vi "Clear_Info.vi"(8 "error in (no error)":errorcluster, 11 "Class in":refnum<class "IB_MSI.lvclass">) -> (0 "error out":errorcluster, 3 "Class out":refnum<class "IB_MSI.lvclass">)   [LabVIEW 2020, in "IB_MSI.lvclass"]
uses:
  <vilib>/AppBuilder/IB_Classes/MSI/IB_MSI.lvclass
  <vilib>/AppBuilder/IB_Classes/MSI/IB_MSI.lvclass/IB_MSI.ctl
  <vilib>/AppBuilder/IB_RW_Project/IB_RW_Project_PropBag_Action.ctl
  <vilib>/AppBuilder/IB_Classes/Installer/Installer.lvclass
  e:/builds/penguin/labview/branches/2020/dev/dist/vi.lib/AppBuilder/IB_Classes/Installer/Installer.lvclass
  e:/builds/penguin/labview/branches/2020/dev/dist/vi.lib/AppBuilder/IB_Classes/MSI/IB_MSI.lvclass
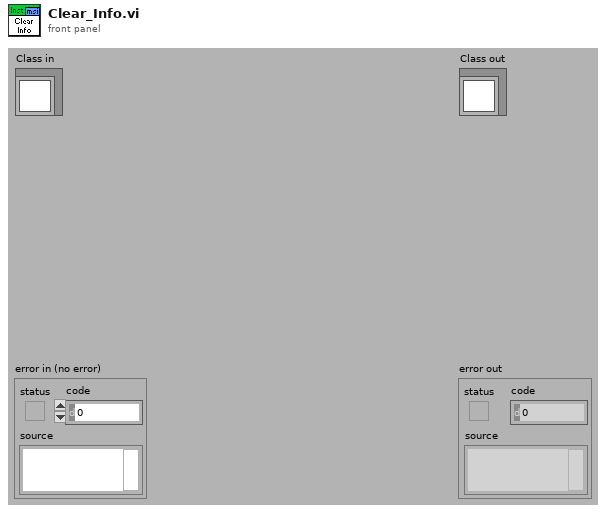
[diagram p1: front panel]
types:
  T1 = typedef "IB_RW_Project_PropBag_Action.ctl" = enum16{"read", "write", "clear", "readPrevious", "writePrevious", "clearPrevious"}
  T2 = typedef "IB_Installer.ctl" = cluster{"Destination":refnum<class "IB_Destination.lvclass">[], "Source":refnum<class "IB_Source.lvclass">[], "buildObject":T3, "defaultDir":string, "platform":string, "author":string, "productName":string, "buildSpecName":string, "hide":bool, "requireLVDevSys":bool, "autoIncrement":bool, "includeError":bool, "readmeID":string, "buildLocation":path, "readmePath":path, "mediaSize":u16, "language":T4, "productVersion":T5, "preview":bool, "programmatic":bool, "progressBarEvents":T6, "userLog_Path":path, "shortcutAddresses":T8[], "EXE_Install Address":string, "EXE_Uninstall Address":string, "additional NIPaths":refnum<class "Dest_NI_NIPath.lvclass">[], "web service itemIDs":string[], "installerName":string}
  T3 = typedef "ItemRef.ctl" = u64
  T4 = typedef "CDK_sTypeDef_Languages.ctl" = u16
  T5 = typedef "CDK_sTypeDef_ProductVersion.ctl" = cluster{"Major":u8, "Minor":u8, "Update":u16}
  T6 = typedef "provcom_ProgressBar_Events.ctl" = cluster{"newJob":refnum<user-event>, "newItem":refnum<user-event>, "errorMsg":T7, "cancel":refnum<user-event>}
  T7 = typedef "mxLvBuildError.ctl" = refnum<user-event>
  T8 = typedef "CDK_sTypeDef_ShortcutAddress.ctl" = cluster{"file":string, "shortcut":string}
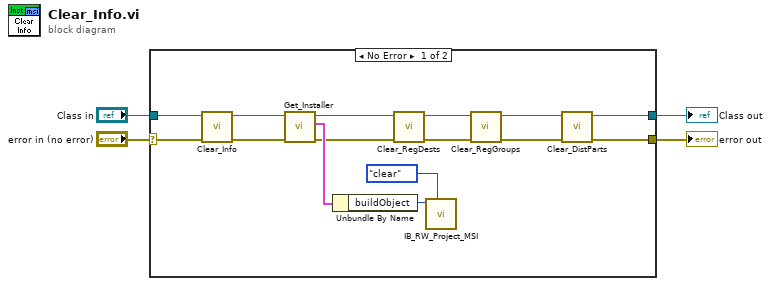
[diagram p0: block diagram]
diagram:
  n1 = case shown="No Error" "error in (no error)" {
    selector: "error in (no error)" -> [w14 w20]
    tunnel: [w9 w20] -> w4
    tunnel: [w10 w21] -> w3
    tunnel: "Class in" -> [w11 w21]
    frame No Error {
      n2 = call-parent "Clear_Info.vi"("error in (no error)"=w14, "Class in"=w11) -> ("error out"=w13:errorcluster, "Class out"=w12:refnum<class "IB_MSI.lvclass">)  [unwired: 8 in]
      n3 = call <vilib>:"Get_Installer.vi"("error in (no error)"=w13, "Installer in"=w12) -> ("error out"=w15:errorcluster, "data"=w18:T2, "Installer out"=w16:refnum<class "IB_MSI.lvclass">)  [unwired: 7 in]
      n4 = Unbundle By Name(w18) -> ("buildObject"=w19:T3)
      n5 = call <vilib>:"Clear_RegDests.vi"("error in (no error)"=w15, "Class in"=w16) -> ("error out"=w6:errorcluster, "Class out"=w8:refnum<class "IB_MSI.lvclass">)  [unwired: 8 in]
      n6 = call <vilib>:"IB_RW_Project_MSI.vi"("action"=IB_RW_Project_PropBag_Action."clear", "Object In"=w19) -> ()  [unwired: 3 in, 7 out]
      n7 = call <vilib>:"Clear_RegGroups.vi"("error in (no error)"=w6, "IB_MSI in"=w8) -> ("error out"=w5:errorcluster, "IB_MSI out"=w7:refnum<class "IB_MSI.lvclass">)  [unwired: 8 in]
      n8 = call <vilib>:"Clear_DistParts.vi"("error in (no error)"=w5, "Class in"=w7) -> ("error out"=w9:errorcluster, "Class out"=w10:refnum<class "IB_MSI.lvclass">)  [unwired: 8 in]
    }
    frame Error {
    }
  }
  "error out" <- w4
  "Class out" <- w3
